vi "upload_ingest.csv.vi"(4 "Properties":map{string, string}(c390), 6 "Labels":string[](array[string]), 7 "Timestamp SeriesName":string, 8 "error in":errorcluster, 9 "timeout (ms)":i32=300000, 10 "File Path":path, 11 "Nominal Client in":refnum<class "Nominal Client.lvclass">) -> (0 "error out":errorcluster, 2 "datasetRID":string, 3 "Nominal Client out":refnum<class "Nominal Client.lvclass">)   [LabVIEW 2020, in "Nominal Client.lvclass"]
doc: "Uploads a file to S3\nIngests video with common settings:\n - No TimeManifest (uses Start Timestamp and a scale factor of 1.\nNew Target: Name based on path name and timestamp"
uses:
  Nominal Client.lvclass
  datasources/dataset/dataset.lvclass
  nominal types/channelConfig/channelConfig.lvclass
  datasources/s3/s3.lvclass
  C:/sw/labview-client/lv_src/datasources/source/source.lvclass
  Nominal Client.lvclass/Nominal Client.ctl
  datasources/target/target.lvclass
  datasources/source/source.lvclass
  datasources/target/create_new.vi
  datasources/source/create_s3.vi
  ingest_csv.vi
  timestampMetadata/timestampMetadata.lvclass
  ts.iso8601/build.iso8601.vi
  ts.iso8601/ts.iso8601.lvclass
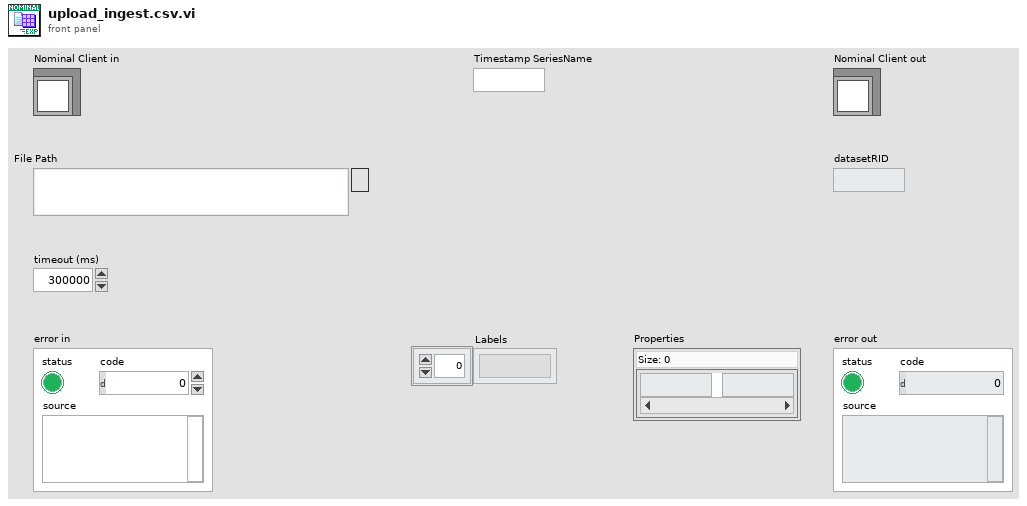
[diagram p1: front panel]
types:
  T1 = cluster{"dataset":refnum<class "dataset.lvclass">, "channelConfig":refnum<class "channelConfig.lvclass">}
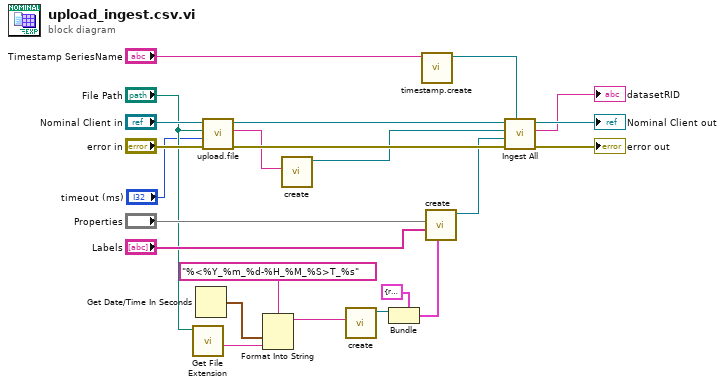
[diagram p0: block diagram]
diagram:
  n1 = call <vilib>:"Get File Extension.vi"("file"="File Path") -> ("filename without extension"=w7:string)  [unwired: 6 in, 4 out]
  n2 = Get Date/Time In Seconds() -> (seconds since 1Jan1904=w2:timestamp)
  n3 = call "upload.file.vi"("error in"="error in", "timeout (ms)"="timeout (ms)", "File"="File Path", "Nominal Client in"="Nominal Client in") -> ("error out"=w22:errorcluster, "Path to S3 File"=w20:string, "Nominal Client out"=w23:refnum<class "Nominal Client.lvclass">)  [unwired: 5 in]
  n4 = Format Into String(format string="%<%Y_%m_%d-%H_%M_%S>T_%s", w2, w7) -> (resulting string=w6:string)  [unwired: 2 in, 1 out]
  n5 = call-poly "create.vi"("Path"=w20) -> ("source"=w19:refnum<class "s3.lvclass">)  [unwired: 10 in]
  n6 = call "create.vi"("Name"=w6) -> ("dataset"=w17:refnum<class "dataset.lvclass">)  [unwired: 10 in]
  n7 = Bundle(cluster=T1 {"dataset"=refnum, "channelConfig"=refnum} ("Optional"), "dataset"=w17) -> (w16:T1)  [unwired: 1 in]
  n8 = call-poly "timestamp.create.vi"("seriesName"="Timestamp SeriesName") -> ("Timestamp Metadata"=w4:refnum<class "timestampMetadata.lvclass">)  [unwired: 10 in]
  n9 = call-poly "create.vi"("Optional"=w16, "Labels"="Labels", "Properties"="Properties") -> ("New Target"=w21:refnum<class "target.lvclass">)  [unwired: 8 in]
  n10 = call-poly "Ingest All.vi"("timestampMetadata"=w4, "error in"=w22, "Target"=w21, "Source"=w19, "Nominal Client in"=w23) -> ("error out"=→"error out":errorcluster, "datasetRid"=→"datasetRID":string, "Nominal Client out"=→"Nominal Client out":refnum<class "Nominal Client.lvclass">)  [unwired: 2 in, 2 out]
